vi "Build Server.vi"(8 "Error In":errorcluster, 10 "Lines":T1[](array[typedef]) {"OPC UA Data Type" items=["Boolean"=1, "SByte"=2, "Byte"=3, "Int16"=4, "UInt16"=5, "Int32"=6, "UInt32"=7, "Int64"=8, "UInt64"=9, "Float"=10, "Double"=11, "String"=12, "DateTime"=13, "ByteString"=15, "Array of Boolean"=101, "Array of SByte"=102, "Array of Byte"=103, "Array of Int16"=104, "Array of UInt16"=105, "Array of Int32"=106, "Array of UInt32"=107, "Array of Int64"=108, "Array of UInt64"=109, "Array of Float"=110, "Array of Double"=111, "Array of String"=112, "Array of DateTime"=113, "Array of ByteString"=115]}, 11 "OPC UA server refnum in":refnum<k21>) -> (0 "Error Out":errorcluster, 3 "OPC UA server refnum out":refnum<k21>)   [LabVIEW 2013, in "OPC UA runtime.lvclass"]
doc: "Build OPC UA Server Folder/Item Hierarchy"
uses:
  OPC UA runtime.lvclass
  configuration/Line.ctl
  <vilib>/NI/Tag Bus Module Framework/channel/TBM channel.lvclass
  configuration/OPC UA Data Type.ctl
  <vilib>/opcua/NI OPC UA Server.lvlib
  configuration/OPC UA configuration.lvclass
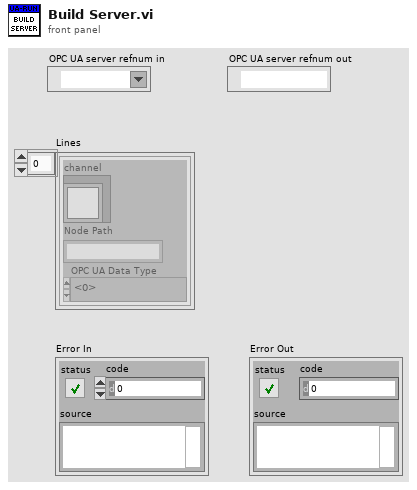
[diagram p1: front panel]
types:
  T1 = typedef "OPC UA configuration.lvclass/Line.ctl" = cluster{"channel":refnum<class "TBM channel.lvclass">, "Node Path":string, "OPC UA Data Type":T2}
  T2 = typedef "OPC UA configuration.lvclass/OPC UA Data Type.ctl" = u16
  T3 = cluster{"name":string, "data type":u16, "access level":u16, "description":string}
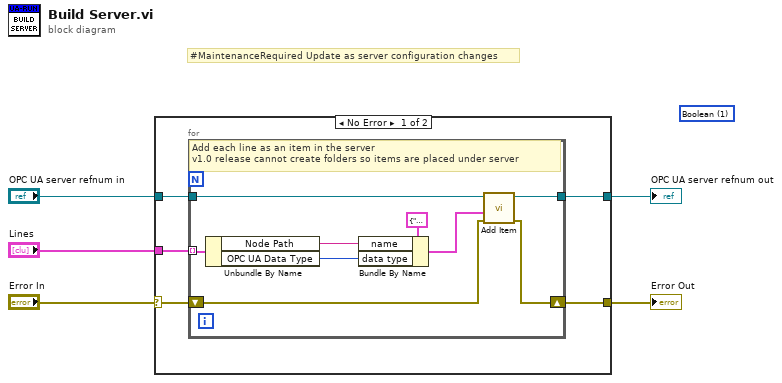
[diagram p0: block diagram]
diagram:
  (unwired) u16 1 items=["Boolean"=1, "SByte"=2, "Byte"=3, "Int16"=4, "UInt16"=5, "Int32"=6, "UInt32"=7, "Int64"=8, "UInt64"=9, "Float"=10, "Double"=11, "String"=12, "DateTime"=13, "ByteString"=15, "Array of Boolean"=101, "Array of SByte"=102, "Array of Byte"=103, "Array of Int16"=104, "Array of UInt16"=105, "Array of Int32"=106, "Array of UInt32"=107, "Array of Int64"=108, "Array of UInt64"=109, "Array of Float"=110, "Array of Double"=111, "Array of String"=112, "Array of DateTime"=113, "Array of ByteString"=115] ("data type")
  # "#MaintenanceRequired Update as server configuration changes"
  n1 = case shown="No Error" "Error In" {
    selector: "Error In" -> [w7 w21]
    tunnel: "OPC UA server refnum in" -> [w10 w20]
    tunnel: "Lines" -> [w9 _]
    tunnel: [w8 w21] -> w3
    tunnel: [w6 w20] -> w1
    frame No Error {
      n2 = for {
        tunnel: w10 -> [w19]
        tunnel: w9 -> [w18] mode=indexing
        shift-right: [w13] -> w8
        shift-left: w7 -> [w14]
        tunnel: [w12] -> w6
        # "Add each line as an item in the server\nv1.0 release cannot create folders so items are placed under server"
        n3 = Unbundle By Name(w18) -> ("Node Path"=w16:string, "OPC UA Data Type"=w11:T2)
        n4 = Bundle By Name(cluster=T3 {"name"="", "data type"=1, "access level"=1, "description"=""} ("item"), "name"=w16, "data type"=w11) -> (w15:T3)
        n5 = call <vilib>:"Add Item.vi"("error in (no error)"=w14, "item"=w15, "OPC UA server refnum in"=w19) -> ("error out"=w13:errorcluster, "OPC UA server refnum out"=w12:refnum<k21>)  [unwired: 5 in, 1 out]
      }
    }
    frame Error {
    }
  }
  "OPC UA server refnum out" <- w1
  "Error Out" <- w3
